vi "Intake_Set.vi"   [LabVIEW 2019]
uses:
  Intake_Cluster.ctl
  Intake_States.ctl
  <vilib>/Rock Robotics/WPI/DriverStation/WPI_DriverStationRobotMode2.ctl
  Globals/Intake_Globals.vi
  Robot Global Data.vi
types:
  T1 = typedef "Intake_Cluster.ctl" = cluster{"Control_State":T2, "Intake_On":bool, "Intake_Extended":bool, "Intake_Throttle":dbl, "Auto_Notifier":refnum<notifier>, "Parameter_1":dbl, "Parameter_2":dbl, "Step":dbl, "Outtake":bool}
  T2 = typedef "Intake_States.ctl" = enum16{"Manual_Throttle", "Manual_Single_Speed", "Compliant_Intake", "Command_RunIntake"}
  T3 = typedef "WPI_DriverStationRobotMode2.ctl" = enum16{"Autonomous Disabled", "Autonomous Enabled", "Teleop Disabled", "Teleop Enabled", "Disconnected", "Finish", "Test Disabled", "Test Enabled", "Emergency Stopped"}
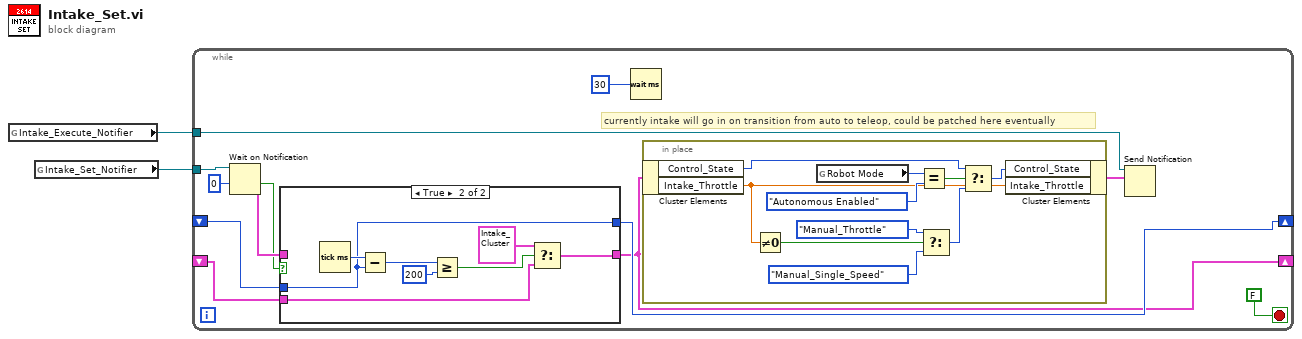
[diagram p0: block diagram]
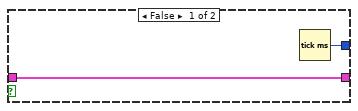
[diagram p2: hidden frame]
diagram:
  n1 = global read "Intake_Globals.vi" "Intake_Execute_Notifier"() -> (w1:refnum<notifier>)
  n2 = global read "Intake_Globals.vi" "Intake_Set_Notifier"() -> (w2:refnum<notifier>)
  n3 = while {
    tunnel: w2 -> [w13]
    tunnel: w1 -> [w12]
    shift-right: [w3] -> _
    shift-left: _ -> [w6]
    shift-right: [w4] -> _
    shift-left: _ -> [w5]
    stop <- FALSE stop-if-true
    # "currently intake will go in on transition from auto to teleop, could be patched here eventually"
    n4 = Wait on Notification(notifier=w13, timeout in ms (-1)=0) -> (notification=w9:T1, timed out?=w8:bool)  [unwired: 2 in, 2 out]
    n5 = case shown="True" w8 {
      tunnel: w9 -> [w16 _]
      tunnel: [w16 w24] -> w3
      tunnel: w6 -> [_ w23]
      tunnel: [w15 w21] -> w4
      tunnel: w5 -> [_ w21]
      frame False {
        n6 = Tick Count (ms)() -> (millisecond timer value=w15:u32)
      }
      frame True {
        n7 = Tick Count (ms)() -> (millisecond timer value=w22:u32)
        n8 = Subtract(x=w22, y=w21) -> (x-y=w19:u32)
        n9 = Greater Or Equal?(x=w19, y=u32 200) -> (x >= y?=w20:bool)
        n10 = Select(t=T1 {"Control_State"=enum."Manual_Throttle", "Intake_On"=FALSE, "Intake_Extended"=FALSE, "Intake_Throttle"=0.0, "Auto_Notifier"=refnum, "Parameter_1"=0.0, "Parameter_2"=0.0, "Step"=0.0, "Outtake"=FALSE}, s=w20, f=w23) -> (s? t:f=w24:T1)
      }
    }
    n11 = Wait (ms)(milliseconds to wait=u32 30) -> ()  [unwired: 1 out]
    n12 = in-place {
      n13 = in-place-cluster #1(w3) -> ("Control_State"=w30:T2, "Intake_Throttle"=w25:dbl)
      n14 = Not Equal To 0?(x=w25) -> (x != 0?=w27:bool)
      n15 = global read "Robot Global Data.vi" "Robot Mode"() -> (w33:T3)
      n16 = Equal?(x=w33, y=WPI_DriverStationRobotMode2."Autonomous Enabled") -> (x = y?=w31:bool)
      n17 = Select(t=Intake_States."Manual_Throttle" ("Control_State"), s=w27, f=Intake_States."Manual_Single_Speed") -> (s? t:f=w29:T2)
      n18 = Select(t=w30, s=w31, f=w29) -> (s? t:f=w34:T2)
      n19 = in-place-cluster #1("Control_State"=w34, "Intake_Throttle"=w25) -> (w11:T1)
    }
    n20 = Send Notification(notification=w11, notifier=w12) -> ()  [unwired: 1 in, 2 out]
  }
